vi "test_MultipleSessionsReserved_InitializeSession_NothingAddedToConnectionMap.vi"(8 "error in":errorcluster) -> (0 "error out":errorcluster, 2 "result":string, 3 "pass":bool)   [LabVIEW 2020, in "MeasurementServerTests.lvlib"]
uses:
  MeasurementServerTests.lvlib
  Helpers/Fake Session Factory/Fake Session Factory.lvclass
  a956f7ee-c7e9-4639-884c-f4265dae6ecf.vi
  Runtime/Measurement Plugin Session Management V1/Session Reservation/Connection.ctl
  Runtime/Measurement Plugin Session Management V1/Session Reservation/Session Reservation.lvclass
  Runtime/Measurement Plugin Session Management V1/Session Reservation/Connection with Session.ctl
  Runtime/Measurement Plugin Measurement Server/Helpers/Error Strings Global Internal.vi
  da202071-85ff-4e27-b7cd-0a9c854c86e4.vi
  Runtime/Measurement Plugin Session Management V1/Session Reservation/Pin Type.ctl
  Runtime/Measurement Plugin Session Management V1/Session Reservation/Initialize and Close Session Behavior.ctl
  48e38c09-e707-4704-822c-9eee424313bf.vi
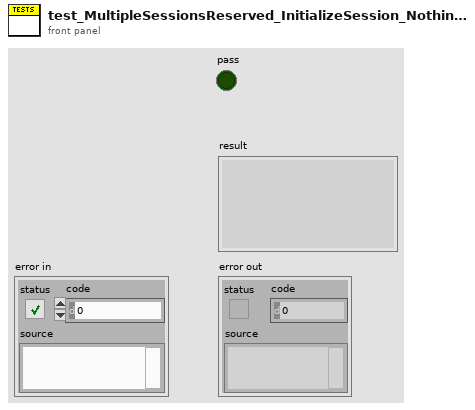
[diagram p1: front panel]
types:
  T1 = typedef "Measurement Plugin Session Management V1.lvlib/Session Reservation.lvclass/Initialize and Close Session Behavior.ctl" = enum16{"Auto", "Initialize and Close", "Attach and Detach", "Initialize and Detach", "Attach and Close"}
  T2 = typedef "Measurement Plugin Session Management V1.lvlib/Session Reservation.lvclass/Pin Type.ctl" = enum16{"DUT and System Pins", "System Pins"}
  T3 = typedef "Measurement Plugin Session Management V1.lvlib/Session Reservation.lvclass/Connection with Session.ctl" = cluster{"connection":T4, "session":variant}
  T4 = typedef "Measurement Plugin Session Management V1.lvlib/Session Reservation.lvclass/Connection.ctl" = cluster{"pin or relay name":string, "site":i32, "instrument type id":string, "channel":string}
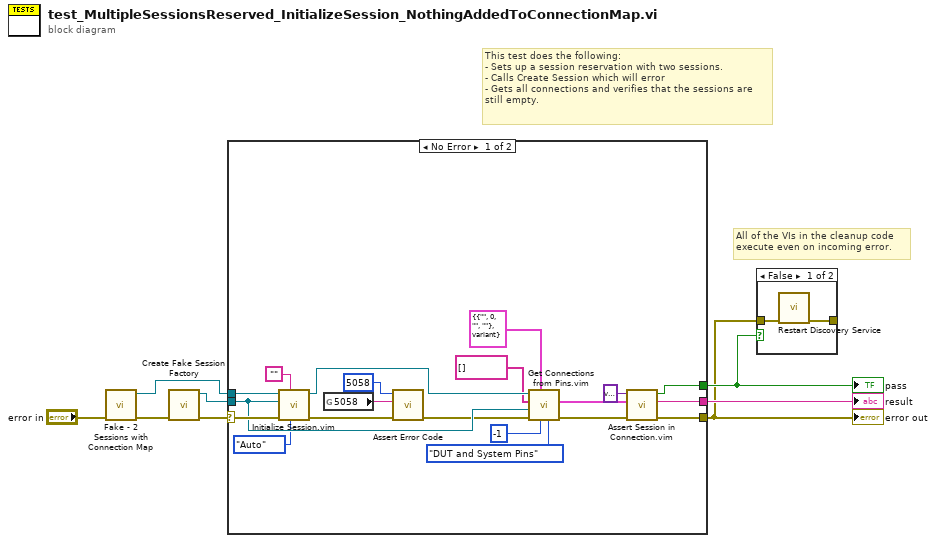
[diagram p0: block diagram]
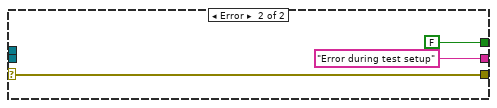
[diagram p2: hidden frame]
diagram:
  # "All of the VIs in the cleanup code\nexecute even on incoming error."
  # "This test does the following:\n- Sets up a session reservation with two sessions.\n- Calls Create Session which will error \n- Gets all connections and verifies that the sessions are\nstill empty."
  n1 = call "Fake - 2 Sessions with Connection Map.vi"("error in"="error in") -> ("error out"=w2:errorcluster, "session reservation out"=w1:refnum<class "Session Reservation.lvclass">)  [unwired: 9 in]
  n2 = call "Create Fake Session Factory.vi"("error in"=w2) -> ("error out"=w5:errorcluster, "fake session factory out"=w4:refnum<class "Fake Session Factory.lvclass">)  [unwired: 9 in]
  n3 = case shown="No Error" w5 {
    selector: w5 -> [w26 w28]
    tunnel: [w19 w28] -> w6
    tunnel: [w12 FALSE] -> w7
    tunnel: [w11 "Error during test setup" ("f")] -> w8
    tunnel: w4 -> [w22 _]
    tunnel: w1 -> [w27 _]
    frame No Error {
      n4 = call "Initialize Session.vim"("initialize and close session behavior"=Initialize_and_Close_Session_Behavior."Auto", "session type"="", "error in"=w26, "session factory"=w22, "session reservation in"=w27) -> ("error out"=w18:errorcluster, "session reservation out"=w24:refnum<class "Session Reservation.lvclass">)  [unwired: 3 in, 2 out]
      n5 = global read "Error Strings Global Internal.vi" "5058"() -> (w16:string)
      n6 = call "Assert Error Code.vi"("error in"=w18, "expected error description"=w16, "expected error code"=5058) -> ("error out"=w17:errorcluster)  [unwired: 6 in, 2 out]
      n7 = call "Get Connections from Pins.vim"("pin type"=Pin_Type."DUT and System Pins", "site"=-1, "connection type"=T3 {"connection"={"pin or relay name"="", "site"=0, "instrument type id"="", "channel"=""}, "session"=variant}, "error in"=w17, "session factory"=w22, "pin or relay names"=string[] [], "session reservation in"=w24) -> ("error out"=w19:errorcluster, "connections"=w14:T3[])  [unwired: 2 in, 1 out]
      n8 = call "Assert Session in Connection.vim"("actual connections"=w14, "expected session"=variant) -> ("result"=w11:string, "pass"=w12:bool)  [unwired: 8 in]
    }
    frame Error {
    }
  }
  "error out" <- w6
  "pass" <- w7
  "result" <- w8
  n9 = case shown="False" w7 {
    tunnel: w6 -> [w32 _]
    tunnel: [w31 _] -> _
    frame False {
      n10 = call "Restart Discovery Service.vi"("error in"=w32) -> ("error out"=w31:errorcluster)  [unwired: 10 in]
    }
    frame True {
    }
  }
